vi "GenArrayIndicesCombination.vi"(11 "Dimension Array":u32[](array[numeric])=[2, 5] caption="Numeric") -> (3 "Index Combinations":string[](array[string])=["[0][0]", "[0][1]", "[0][2]", "[0][3]", "[0][4]", "[1][0]", "[1][1]", "[1][2]", "[1][3]", "[1][4]"])   [LabVIEW 2015, in "LVdataToTableData.lvlib"]
uses:
  LVdataToTableData/LVdataToTableData.lvlib
panel:
  # "Connector Pane"
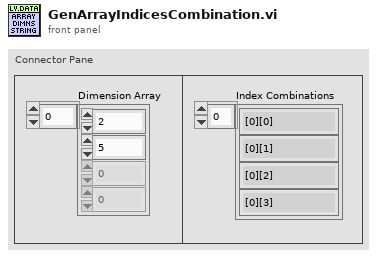
[diagram p1: front panel]
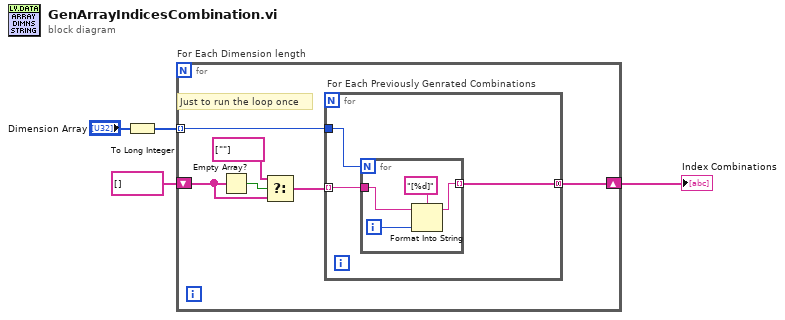
[diagram p0: block diagram]
diagram:
  n1 = To Long Integer(number="Dimension Array") -> (32bit integer=w1:i32[])
  n2 = for "For Each Dimension length" {
    tunnel: w1 -> [w7] mode=indexing
    shift-right: [w6] -> w2
    shift-left: string[] [] ("Array") -> [w10]
    # "Just to run the loop once"
    n3 = Empty Array?(array=w10) -> (empty?=w5:bool)
    n4 = Select(t=string[] [""], s=w5, f=w10) -> (s? t:f=w8:string[])
    n5 = for "For Each Previously Genrated Combinations" {
      tunnel: w8 -> [w12] mode=indexing
      tunnel: w7 -> [w13]
      tunnel: [w11] -> w6 mode=concatenating
      n6 = for {
        N: w13 -> [_]
        tunnel: [w17] -> w11 mode=indexing
        tunnel: w12 -> [w14]
        i -> [w16]
        n7 = Format Into String(format string="[%d]", initial string=w14, w16) -> (resulting string=w17:string)  [unwired: 1 in, 1 out]
      }
    }
  }
  "Index Combinations" <- w2
